vi "Get Error.vi"(0 "LVx.lvlib:LVx.lvclass":refnum<class "LVx.lvclass">, 11 "error in (no error)":errorcluster) -> (4 "LVx.lvlib:LVx.lvclass 2":refnum<class "LVx.lvclass">, 15 "error out":errorcluster)   [LabVIEW 2011, in "LVx.lvlib" / "LVx.lvclass"]
uses:
  LVx.lvclass
  LVx.lvclass/LVx.ctl
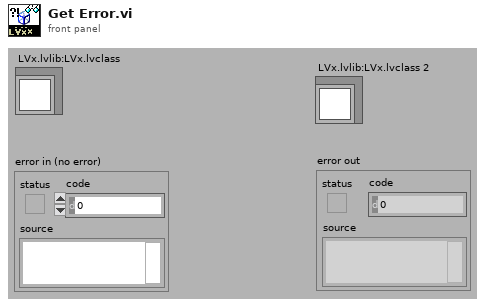
[diagram p1: front panel]
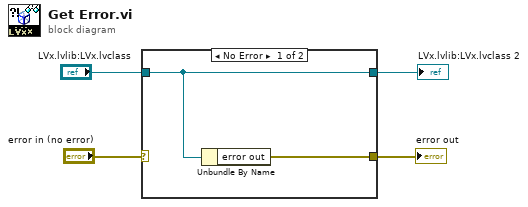
[diagram p0: block diagram]
diagram:
  n1 = case shown="No Error" "error in (no error)" {
    selector: "error in (no error)" -> [_ w8]
    tunnel: "LVx.lvlib:LVx.lvclass" -> [w5 w7]
    tunnel: [w6 w8] -> w3
    tunnel: [w5 w7] -> w1
    frame No Error {
      n2 = Unbundle By Name(w5) -> ("error out"=w6:errorcluster)
    }
    frame Error {
    }
  }
  "error out" <- w3
  "LVx.lvlib:LVx.lvclass 2" <- w1
